vi "Get Property Flags.vi"(8 "error in (no error)":errorcluster, 10 "Property ID":string="2c7a809", 11 "Class ID":string) -> (0 "error out":errorcluster, 3 "Property Flags":T2)   [LabVIEW 2023]
doc: "Sets the class specifier constant on the helper VI and the property of the first property item on the attached property node, and reads off the property flags, R/W status, adn class type if the property returns a reference.\n\n\nIf class type is unqired, the class is unchanged, which may speed up the Get All Properties VI, which has already set the class specifier constant in a prior step.\n\n\n<b> </b> <b> </b>\n© 2017 Q Software Innovations, LLC\nwritten by Quentin \"Q\" Alldredge\nproduced in LabVIEW 2015\n\nsupport@qsoftwareinnovations.com\nwww.qsoftwareinnovations.com\n\nAll rights reserved.\n\nRedistribution and use in source and binary forms, with or without modification, are permitted provided that the following conditions are met:\n\n * Redistributions of source code must retain the above copyright notice, this list of conditions and the following disclaimer.\n * Redistributions in binary form must reproduce the above copyright notice, this list of conditions and the following disclaimer in the documentation and/or other materials provided with the distribution.\n * Neither the name of Q Software Innovations, LLC. nor the names of its contributors may be used to endorse or promote products derived from this software without specific prior written permission.\n\nTHIS SOFTWARE IS PROVIDED BY THE COPYRIGHT HOLDERS AND CONTRIBUTORS \"AS IS\" AND ANY EXPRESS OR IMPLIED WARRANTIES, INCLUDING, BUT NOT LIMITED TO, THE IMPLIED WARRANTIES OF MERCHANTABILITY AND FITNESS FOR A PARTICULAR PURPOSE ARE DISCLAIMED. IN NO EVENT SHALL THE COPYRIGHT OWNER OR CONTRIBUTORS BE LIABLE FOR ANY DIRECT, INDIRECT, INCIDENTAL, SPECIAL, EXEMPLARY, OR CONSEQUENTIAL DAMAGES (INCLUDING, BUT NOT LIMITED TO, PROCUREMENT OF SUBSTITUTE GOODS OR SERVICES; LOSS OF USE, DATA, OR PROFITS; OR BUSINESS INTERRUPTION) HOWEVER CAUSED AND ON ANY THEORY OF LIABILITY, WHETHER IN CONTRACT, STRICT LIABILITY, OR TORT (INCLUDING NEGLIGENCE OR OTHERWISE) ARISING IN ANY WAY OUT OF THE USE OF THIS SOFTWARE, EVEN IF ADVISED OF THE POSSIBILITY OF SUCH DAMAGE."
uses:
  <vilib>/Utility/Data Type/NI_Data Type.lvlib
panel:
  out "type":T1(ring)
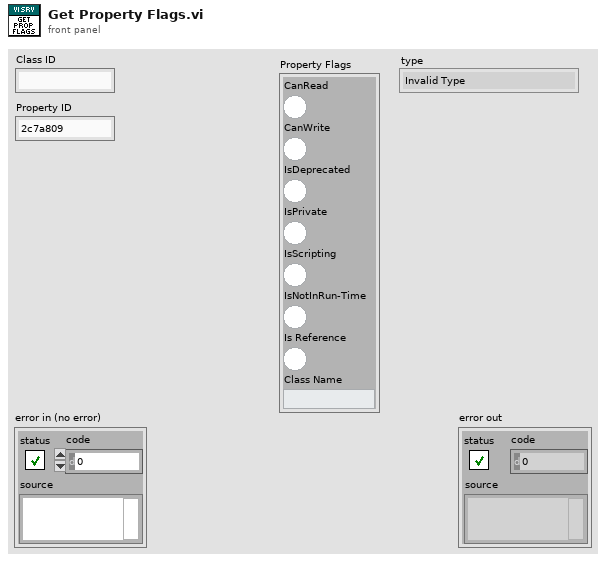
[diagram p1: front panel]
types:
  T1 = enum8{"Invalid Type", "Void", "I8", "I16", "I32", "I64", "U8", "U16", "U32", "U64", "Single Float", "Double Float", "Extended Float", "Single Complex", "Double Complex", "Extended Complex", "Enum U8", "Enum U16", "Enum U32", "Enum U64", "Single Float With Unit", "Double Float With Unit", "Extended Float With Unit", "Single Complex with Unit", "Double Complex with Unit", "Extended Complex with Unit", "Boolean", "String", "Path", "Picture", "Tag", "Array", "Cluster", "Variant", "LV Variant", "Waveform", "Timestamp", "Digital Waveform", "Digital Data", "ExpressData", "Refnum", "External Data", "VI", "Poly VI", "LabVIEW Class Instance", "Fixed Point"}
  T2 = cluster{"CanRead":bool, "CanWrite":bool, "IsDeprecated":bool, "IsPrivate":bool, "IsScripting":bool, "IsNotInRun-Time":bool, "Is Reference":bool, "Class Name":string}
  T3 = typedef "NI_Data Type.lvlib/Data Type.ctl" = enum8{"Invalid Type", "Void", "I8", "I16", "I32", "I64", "U8", "U16", "U32", "U64", "Single Float", "Double Float", "Extended Float", "Single Complex", "Double Complex", "Extended Complex", "Enum U8", "Enum U16", "Enum U32", "Enum U64", "Single Float With Unit", "Double Float With Unit", "Extended Float With Unit", "Single Complex with Unit", "Double Complex with Unit", "Extended Complex with Unit", "Boolean", "String", "Path", "Picture", "Tag", "Array", "Cluster", "Variant", "LV Variant", "Waveform", "Timestamp", "Digital Waveform", "Digital Data", "ExpressData", "Refnum", "External Data", "VI", "Poly VI", "LabVIEW Class Instance", "Fixed Point", "Set Collection", "Map Collection"}
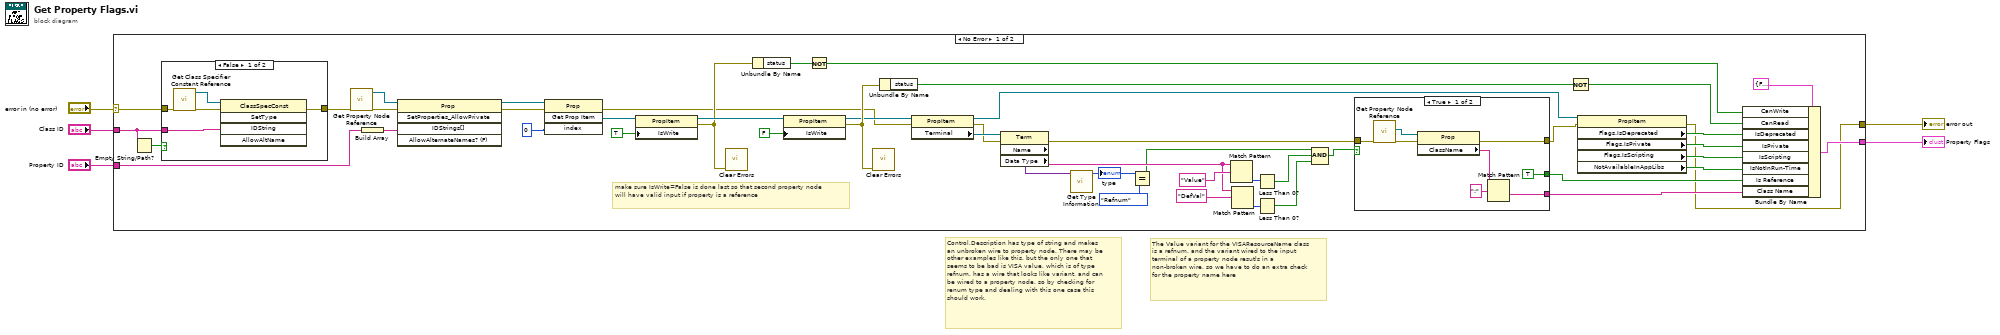
[diagram p0: block diagram]
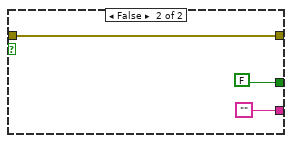
[diagram p3: hidden frame]
diagram:
  # "Control.Description has type of string and makes an unbroken wire to property node. There may be other examples like this, but the only one that seems to be bad is VISA value, which is of type refnum, has a wire that looks like variant, and can be wired to a property node, so by checking for renum type and dealing with this one case this should work."
  # "The Value variant for the VISAResourceName class is a refnum, and the variant wired to the input terminal of a property node resutls in a non-broken wire, so we have to do an extra check for the property name here"
  n1 = case shown="No Error" "error in (no error)" {
    selector: "error in (no error)" -> [w54 w72]
    tunnel: [w19 w72] -> w4
    tunnel: "Class ID" -> [w22 _]
    tunnel: "Property ID" -> [w50 _]
    tunnel: [w46 _] -> w1
    frame No Error {
      # "make sure IsWrite=False is done last so that second property node will have valid input if property is a reference"
      n2 = Empty String/Path?(string/path=w22) -> (empty?=w21:bool)
      n3 = case shown="False" w21 {
        tunnel: w54 -> [w59 w60]
        tunnel: w22 -> [w56 _]
        tunnel: [w55 w60] -> w53
        frame False {
          n4 = call "Get Class Specifier Constant Reference.vi"("error in (no error)"=w59) -> ("error out"=w57:errorcluster, "specific class reference"=w58:refnum<vi>)  [unwired: 9 in]
          n5 = invoke class="ClassSpecConst" method="SetType"(reference=w58, error in=w57, "IDString"=w56) -> (error out=w55:errorcluster)  [unwired: 2 in, 4 out]
        }
        frame True {
        }
      }
      n6 = call "Get Property Node Reference.vi"("error in (no error)"=w53) -> ("error out"=w52:errorcluster, "Main Prop Refnum"=w51:refnum<vi>)  [unwired: 8 in, 1 out]
      n7 = Build Array(w50) -> (w49:string[])
      n8 = invoke class="Prop" method="SetProperties_AllowPrivate"(reference=w51, error in=w52, "IDStrings[]"=w49) -> (reference out=w38:refnum<vi>, error out=w48:errorcluster)  [unwired: 2 in, 3 out]
      n9 = invoke class="Prop" method="Get Prop Item"(reference=w38, error in=w48, "index"=u32 0 ("Index")) -> (error out=w28:errorcluster, "Get Prop Item"=w41:refnum<vi>)  [unwired: 1 in, 2 out]
      n10 = property class="PropItem"(reference=w41, "IsWrite"=TRUE ("Is Write")) -> (reference out=w39:refnum<vi>, error out=w35:errorcluster)  [unwired: 1 in]
      n11 = call <vilib>:"Clear Errors.vi"("error in (no error)"=w35) -> ()  [unwired: 5 in, 2 out]
      n12 = Unbundle By Name(w35) -> ("status"=w34:bool)
      n13 = property class="PropItem"(reference=w39, "IsWrite"=FALSE ("Is Write")) -> (reference out=w29:refnum<vi>, error out=w31:errorcluster)  [unwired: 1 in]
      n14 = Not(x=w34) -> (.not. x?=w33:bool)
      n15 = call <vilib>:"Clear Errors.vi"("error in (no error)"=w31) -> ()  [unwired: 5 in, 2 out]
      n16 = Unbundle By Name(w31) -> ("status"=w32:bool)
      n17 = property class="PropItem"(reference=w29, error in=w28) -> (reference out=w6:refnum<vi>, error out=w26:errorcluster, "Terminal"=w27:refnum<vi>)
      n18 = property class="Term"(reference=w27, error in=w26) -> (error out=w20:errorcluster, "Name"=w14:string, "Data Type"=w10:variant)  [unwired: 1 out]
      n19 = call <vilib>:"Get Type Information.vi"("variant"=w10) -> ("type"=w9:T3)  [unwired: 6 in, 4 out]
      "type" <- w9
      n20 = Equal?(x=w9, y=T1."Refnum") -> (x = y?=w7:bool)
      n21 = Match Pattern(string=w14, regular expression="Value") -> (offset past match=w17:i32)  [unwired: 1 in, 3 out]
      n22 = Match Pattern(string=w14, regular expression="DefVal") -> (offset past match=w13:i32)  [unwired: 1 in, 3 out]
      n23 = Less Than 0?(x=w17) -> (x < 0?=w12:bool)
      n24 = Less Than 0?(x=w13) -> (x < 0?=w11:bool)
      n25 = Compound Arithmetic op=AND(w7, w12, w11) -> (w16:bool)
      n26 = case shown="True" w16 {
        tunnel: w20 -> [w67 w71]
        tunnel: [w65 w71] -> w25
        tunnel: [w62 ""] -> w24
        tunnel: [TRUE FALSE] -> w23
        frame True {
          n27 = call "Get Property Node Reference.vi"("error in (no error)"=w67) -> ("error out"=w66:errorcluster, "Secondary Prop Refnum"=w68:refnum<vi>)  [unwired: 8 in, 1 out]
          n28 = property class="Prop"(reference=w68, error in=w66) -> (error out=w65:errorcluster, "ClassName"=w63:string)  [unwired: 1 out]
          n29 = Match Pattern(string=w63, regular expression=":") -> (after substring=w62:string)  [unwired: 1 in, 3 out]
        }
        frame False {
        }
      }
      n30 = Not(x=w32) -> (.not. x?=w30:bool)
      n31 = property class="PropItem"(reference=w6, error in=w25) -> (error out=w19:errorcluster, "Flags.IsDeprecated"=w43:bool, "Flags.IsPrivate"=w44:bool, "Flags.IsScripting"=w45:bool, "NotAvailableInAppLibs"=w37:bool)  [unwired: 1 out]
      n32 = Bundle By Name(cluster=T2 {"CanRead"=FALSE, "CanWrite"=FALSE, "IsDeprecated"=FALSE, "IsPrivate"=FALSE, "IsScripting"=FALSE, "IsNotInRun-Time"=FALSE, "Is Reference"=FALSE, "Class Name"=""}, "CanWrite"=w33, "CanRead"=w30, "IsDeprecated"=w43, "IsPrivate"=w44, "IsScripting"=w45, "IsNotInRun-Time"=w37, "Is Reference"=w23, "Class Name"=w24) -> (w46:T2)
    }
    frame Error {
    }
  }
  "error out" <- w4
  "Property Flags" <- w1
